vi "AppendTimestamp.vi"(7 "time stamp":timestamp, 10 "String":string) -> (2 "String With Time Added":string)   [LabVIEW 2016]
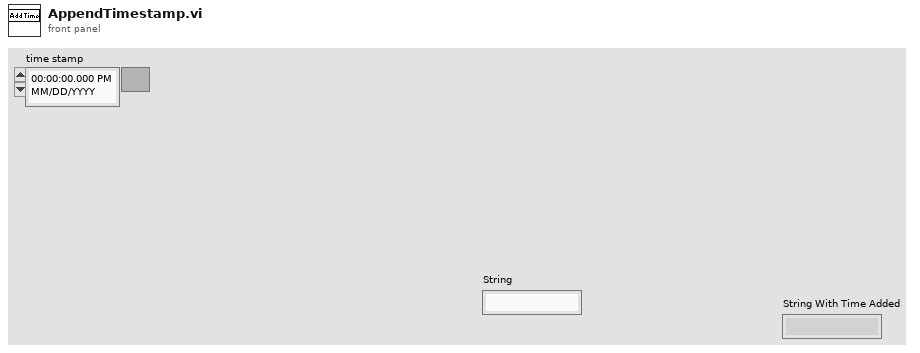
[diagram p1: front panel]
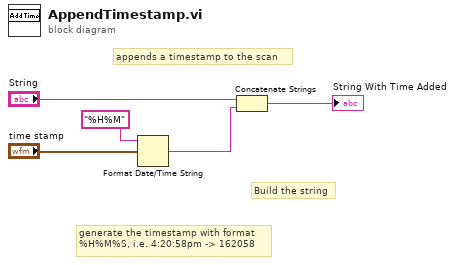
[diagram p0: block diagram]
diagram:
  # "Build the string"
  # "generate the timestamp with format\n%H%M%S, i.e. 4:20:58pm -> 162058"
  # "appends a timestamp to the scan"
  n1 = Format Date/Time String(time format string (%c)="%H%M", seconds (now)="time stamp") -> (date/time string=w3:string)  [unwired: 1 in]
  n2 = Concatenate Strings("String", w3) -> (→"String With Time Added":string)
